vi "PH_gentec_M-Link.Action open connection.vi"(0 "i ref in":refnum<vi>, 2 "VISA resource in":refnum<visa-resource-name>, 5 "error in":errorcluster) -> (14 "i ref out":refnum<vi>, 19 "error out":errorcluster)   [LabVIEW 2014, in "PH_gentec_M-Link.lvlib"]
doc: "This VI opens the VISA connection."
uses:
  PH_gentec_M-Link.lvlib
  PH_Basics/PH_Powermeter_BaseClass/PH_Powermeter_BaseClass.State.ctl
  PH_Basics/PH_Powermeter_BaseClass/PH_Powermeter_BaseClass.Connection.ctl
  instr.lib/Gentec-M-Link/gentec-M-Link - Driver.lvlib
  PH_Basics/PH_Powermeter_BaseClass/PH_Powermeter_BaseClass.lvlib
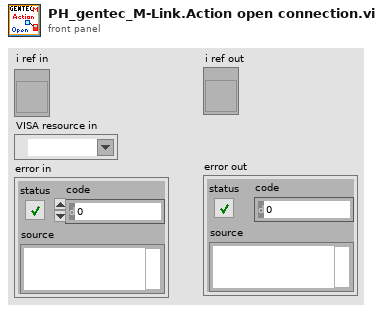
[diagram p1: front panel]
types:
  T1 = typedef "PH_Powermeter_BaseClass.lvlib/PH_Powermeter_BaseClass.Connection.ctl" = cluster{"failed checks":i8, "Timeout":bool, "Data read":string, "Failure":bool, "Error":bool, "State":T2}
  T2 = typedef "PH_Powermeter_BaseClass.lvlib/PH_Powermeter_BaseClass.State.ctl" = enum32{"off", "operating", "opened", "checked", "connected", "Sets to change", "running"}
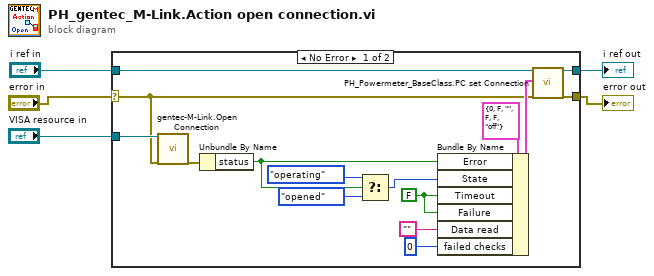
[diagram p0: block diagram]
diagram:
  n1 = case shown="No Error" "error in" {
    selector: "error in" -> [w7 w22]
    tunnel: [w6 w22] -> w5
    tunnel: "VISA resource in" -> [w18 _]
    tunnel: "i ref in" -> [w11 w21]
    tunnel: [w8 w21] -> w1
    frame No Error {
      w17 = FALSE ("Connection.Timeout")
      n2 = call "gentec-M-Link.Open Connection.vi"("VISA resource (In)"=w18, "error in (no error)"=w7) -> ("error out"=w19:errorcluster)  [unwired: 16 in, 1 out]
      n3 = Unbundle By Name(w19) -> ("status"=w16:bool)
      n4 = Select(t=PH_Powermeter_BaseClass.State."operating" ("State"), s=w16, f=PH_Powermeter_BaseClass.State."opened") -> (s? t:f=w13:T2)
      n5 = Bundle By Name(cluster=T1 {"failed checks"=0, "Timeout"=FALSE, "Data read"="", "Failure"=FALSE, "Error"=FALSE, "State"=enum."off"} ("Connection in"), "Error"=w16, "State"=w13, "Timeout"=w17, "Failure"=w17, "Data read"="", "failed checks"=i8 0) -> (w9:T1)
      n6 = call "PH_Powermeter_BaseClass.PC set Connection.vi"("VI in"=w11, "Connection"=w9, "error in (no error)"=w7) -> ("VI out"=w8:refnum<vi>, "error out"=w6:errorcluster)  [unwired: 15 in]
    }
    frame Error {
    }
  }
  "error out" <- w5
  "i ref out" <- w1
